vi "reg-status.vi"(6 "Operation(Read)":T1, 8 "error in":errorcluster, 11 "Reports to Collect":string) -> (0 "error out":errorcluster, 3 "Collected Reports":string)   [LabVIEW 2024]
uses:
  controls/enum.report-filter.ctl
  <vilib>/Utility/error.llb/Trim Whitespace.vi
  <vilib>/Utility/error.llb/Trim Whitespace One-Sided.vi
panel:
  out "size(s)":i32
  in  "Rows":i32=100
  # "stepIndex>=0 then filter by step index\nstepIndex==-1 then do not filter"
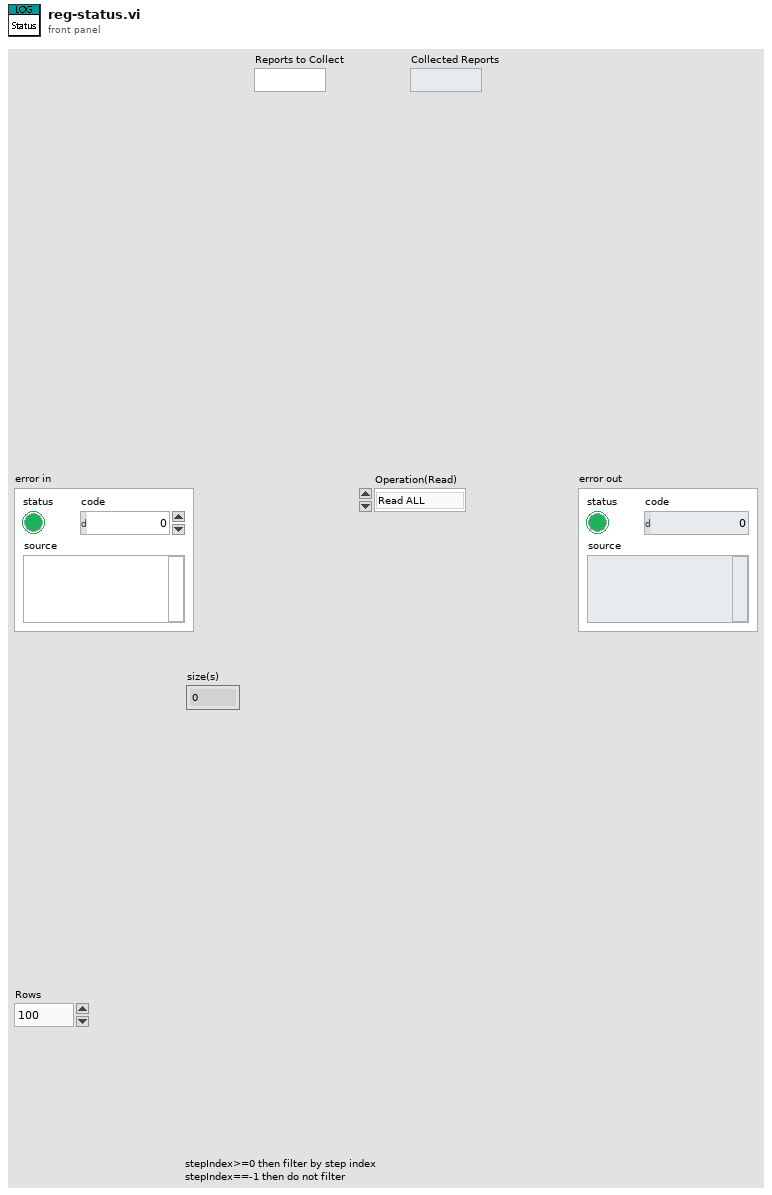
[diagram p1: front panel]
types:
  T1 = typedef "enum.report-filter.ctl" = enum16{"Read ALL", "Read Errors", "Collect", "ClearAll"}
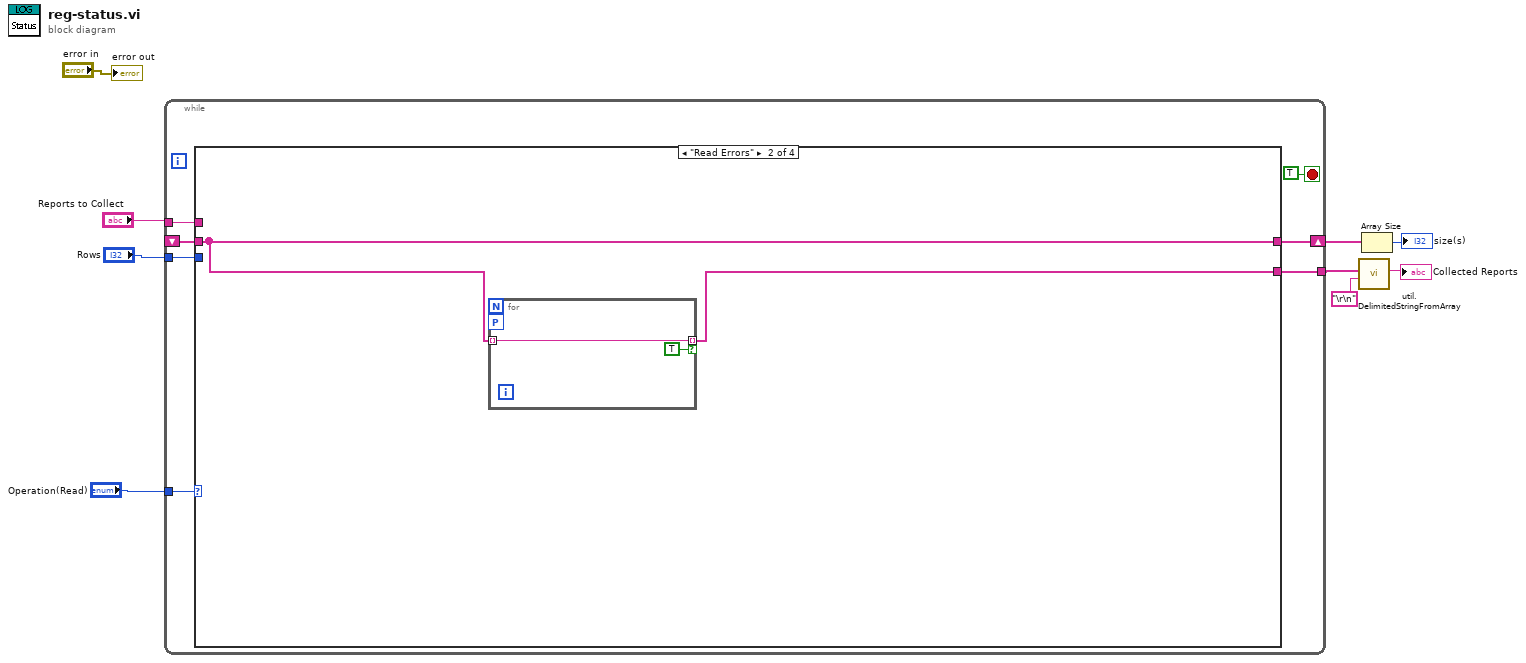
[diagram p0: block diagram]
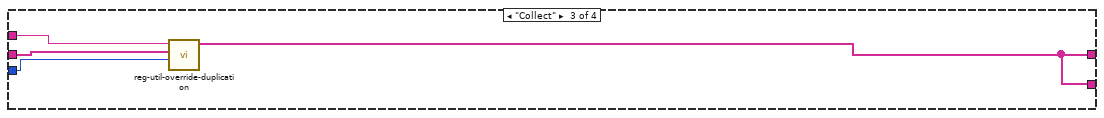
[diagram p3: hidden frame]
diagram:
  n1 = while {
    shift-right: [w14] -> w6
    shift-left: _ -> [w12]
    tunnel: "Reports to Collect" -> [w16]
    tunnel: "Rows" -> [w13]
    tunnel: "Operation(Read)" -> [w11]
    tunnel: [w10] -> w3
    stop <- TRUE stop-if-true
    n2 = case shown="\"Read Errors\"" w11 {
      tunnel: w16 -> [_ _ w25 _]
      tunnel: [w17 w19 w22 _] -> w14
      tunnel: w13 -> [_ _ w23 _]
      tunnel: w12 -> [w17 w19 w24 _]
      tunnel: [w17 w18 w22 _] -> w10
      frame "Read ALL", Default {
      }
      frame "Read Errors" {
        n3 = for {
          tunnel: w19 -> [w21] mode=indexing
          tunnel: [w21] -> w18 mode=indexing if=TRUE
          workers-P: _ -> [_]
        }
      }
      frame "Collect" {
        n4 = call "reg-util-override-duplication.vi"("Rows"=w23, "string register"=w24, "Reports to Collect"=w25) -> ("string register"=w22:string[])  [unwired: 8 in]
      }
      frame "ClearAll" {
      }
    }
  }
  n5 = call "util.DelimitedStringFromArray.vi"("delimiter (Comma)"="\r\n", "params array in"=w3) -> ("delimited string out"=→"Collected Reports":string)  [unwired: 9 in]
  n6 = Array Size(array=w6) -> (size(s)=→"size(s)":i32)
  "error out" <- "error in"
